vi "Ke2400 OPC.vi"(6 "Time Out":u32, 8 "error in (no error)":errorcluster, 11 "VISA resource name":refnum<visa-resource-name>) -> (0 "error out":errorcluster, 3 "VISA Out":refnum<visa-resource-name>)   [LabVIEW 2012]
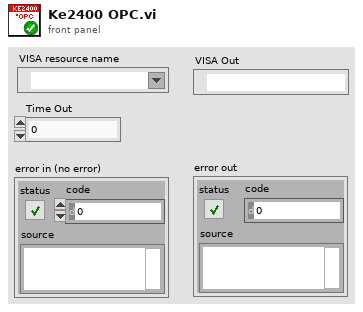
[diagram p1: front panel]
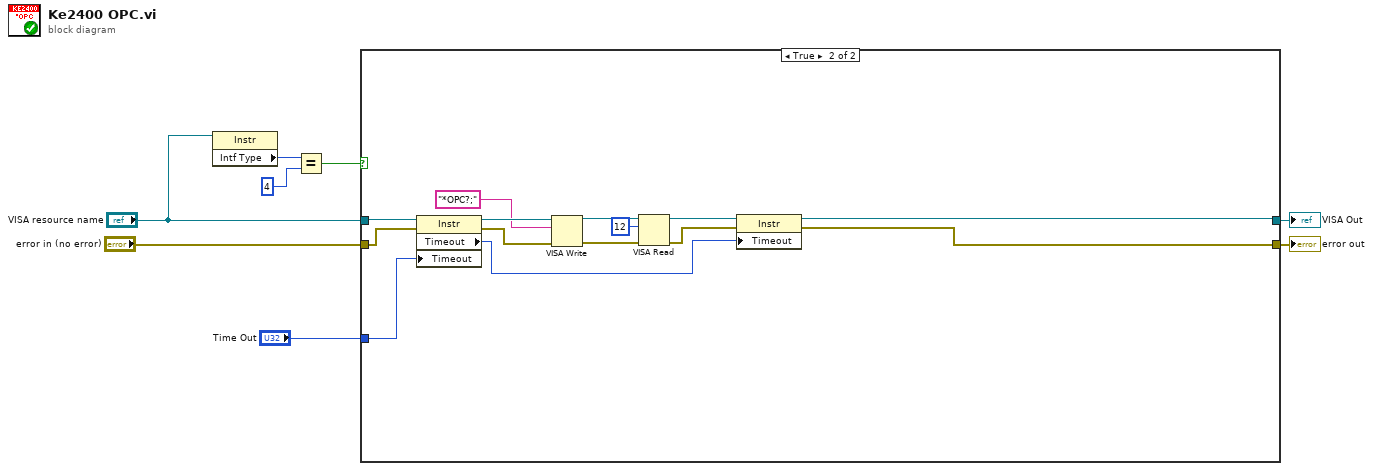
[diagram p0: block diagram]
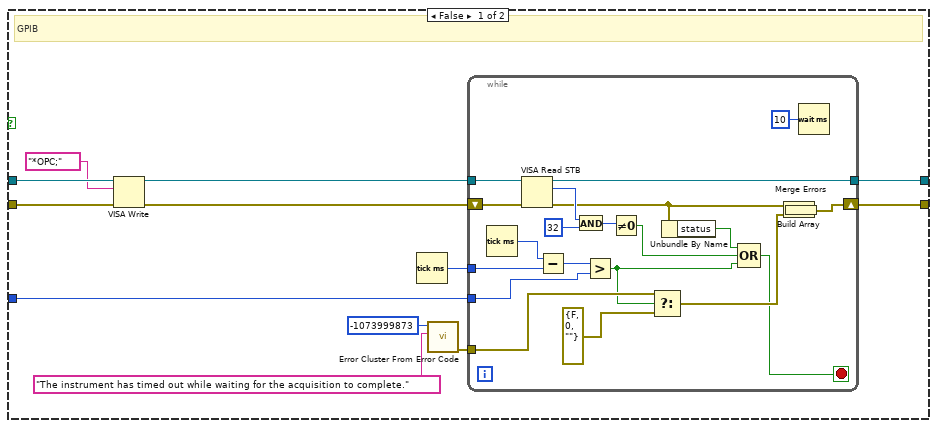
[diagram p2: hidden frame]
diagram:
  n1 = property class="Instr"(reference="VISA resource name") -> ("Intf Type"=w6:u16)  [unwired: 1 in, 2 out]
  n2 = Equal?(x=w6, y=u16 4) -> (x = y?=w4:bool)
  n3 = case shown="True" w4 {
    tunnel: "error in (no error)" -> [w20 w54]
    tunnel: "VISA resource name" -> [w19 w55]
    tunnel: "Time Out" -> [w12 w53]
    tunnel: [w11 w43] -> w2
    tunnel: [w10 w42] -> w1
    frame False {
      # "GPIB"
      n4 = VISA Write(VISA resource name=w19, write buffer="*OPC;", error in (no error)=w20) -> (VISA resource name out=w14:refnum<visa-resource-name>, error out=w16:errorcluster)  [unwired: 1 out]
      n5 = Tick Count (ms)() -> (millisecond timer value=w13:u32)
      n6 = call <vilib>:"Error Cluster From Error Code.vi"("error message (\"\")"="The instrument has timed out while waiting for the acquisition to complete." ("error message (\"\")"), "error code (0)"=-1073999873) -> ("error out"=w15:errorcluster)  [unwired: 7 in]
      n7 = while {
        shift-right: [w35] -> w11
        shift-left: w16 -> [w38]
        tunnel: w15 -> [w41]
        tunnel: w14 -> [w37]
        tunnel: w13 -> [w27]
        tunnel: w12 -> [w25]
        tunnel: [w22] -> w10
        stop <- w23 stop-if-true
        n8 = Tick Count (ms)() -> (millisecond timer value=w28:u32)
        n9 = VISA Read STB(8:w38, 11:w37) -> (0:w30:errorcluster, 2:w36:u16, 3:w22:refnum<visa-resource-name>)
        n10 = Subtract(x=w28, y=w27) -> (x-y=w26:u32)
        n11 = And(x=w36, y=u16 32) -> (x .and. y?=w32:u16)
        n12 = Greater?(x=w26, y=w25) -> (0:w24:bool)
        n13 = Not Equal To 0?(x=w32) -> (x != 0?=w31:bool)
        n14 = Select(t=w41, s=w24, f=errorcluster {"status"=FALSE, "code"=0, "source"=""}) -> (s? t:f=w39:errorcluster)
        n15 = Unbundle By Name(w30) -> ("status"=w29:bool)
        n16 = Compound Arithmetic op=OR(w29, w31, w24) -> (w23:bool)
        n17 = Build Array(w30, w39) -> (w34:errorcluster[])
        n18 = Merge Errors(w34) -> (w35:errorcluster)
        n19 = Wait (ms)(milliseconds to wait=u32 10) -> ()  [unwired: 1 out]
      }
    }
    frame True {
      n20 = property class="Instr"(reference=w55, error in=w54, "Timeout"=w53) -> (reference out=w52:refnum<visa-resource-name>, error out=w51:errorcluster, "Timeout"=w45:u32)
      n21 = VISA Write(VISA resource name=w52, write buffer="*OPC?;", error in (no error)=w51) -> (VISA resource name out=w48:refnum<visa-resource-name>, error out=w49:errorcluster)  [unwired: 1 out]
      n22 = VISA Read(VISA resource name=w48, byte count=u32 12, error in (no error)=w49) -> (VISA resource name out=w46:refnum<visa-resource-name>, error out=w44:errorcluster)  [unwired: 2 out]
      n23 = property class="Instr"(reference=w46, error in=w44, "Timeout"=w45) -> (reference out=w42:refnum<visa-resource-name>, error out=w43:errorcluster)
    }
  }
  "error out" <- w2
  "VISA Out" <- w1
